vi "DM get burst by index.vi"(8 "error in (no error)":errorcluster, 10 "Burst name":i32, 11 "group":string) -> (0 "error out":errorcluster, 3 "TX burst":refnum<class "mmWave data.lvclass">)   [LabVIEW 2019, in "DataManagment.lvlib"]
uses:
  DataManagment.lvlib
  SubVIs/mmWave data_class/mmWave data.lvclass
  DM get burst by index parameters.ctl
  <vilib>/Utility/error.llb/Error Cluster From Error Code.vi
  <vilib>/ErrorRing/Error Ring.xnode
  <vilib>/addons/_JKI.lib/Serialization/JSON/JKI JSON Serialization.lvlib
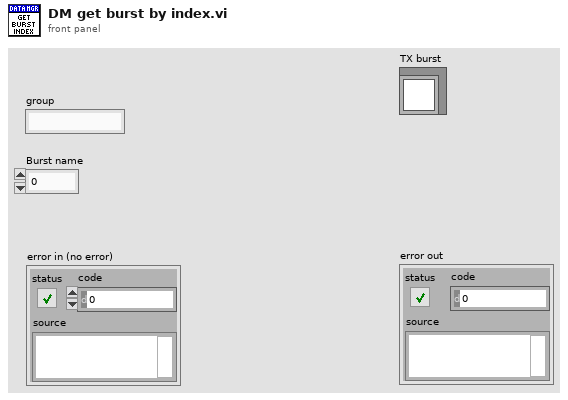
[diagram p1: front panel]
types:
  T1 = typedef "DataManagment.lvlib/DM get burst by index parameters.ctl" = cluster{"group":string, "index":i32}
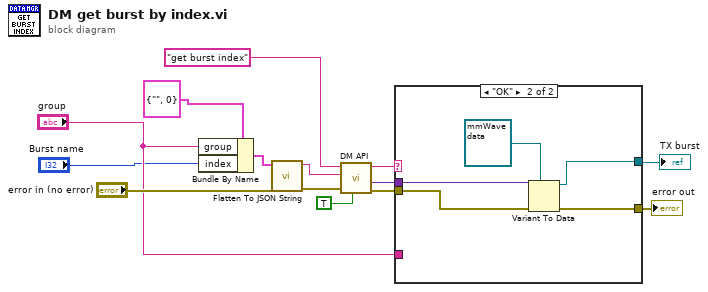
[diagram p0: block diagram]
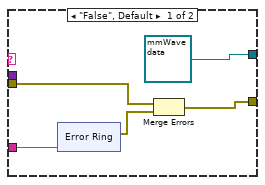
[diagram p2: hidden frame]
diagram:
  n1 = Bundle By Name(cluster=T1 {"group"="", "index"=0} ("Cluster"), "group"="group", "index"="Burst name") -> (w7:T1)
  n2 = call <vilib>:"Flatten To JSON String.vi"("error in (no error)"="error in (no error)", "Variant"=w7) -> ("error out"=w5:errorcluster, "JSON String"=w4:string)  [unwired: 8 in]
  n3 = call "DM API.vi"("response"=TRUE, "error in (no error)"=w5, "parameters"=w4, "message"="get burst index") -> ("error out"=w9:errorcluster, "data"=w11:variant, "status"=w12:string)  [unwired: 4 in, 1 out]
  n4 = case shown="\"OK\"" w12 {
    tunnel: w11 -> [_ w31]
    tunnel: [refnum<class "mmWave data.lvclass"> refnum ("mmWave data") w27] -> w10
    tunnel: [w17 w28] -> w8
    tunnel: w9 -> [w16 w29]
    tunnel: "group" -> [w15 _]
    frame "False", Default {
      n5 = xnode "Error Ring"("parameter 0"=w15) -> ("error out"=w18:errorcluster)
      n6 = Merge Errors(w16, w18) -> (w17:errorcluster)
    }
    frame "OK" {
      n7 = Variant To Data(error in=w29, type=refnum<class "mmWave data.lvclass"> refnum ("Array"), Variant=w31) -> (data=w27:refnum<class "mmWave data.lvclass">, error out=w28:errorcluster)
    }
  }
  "TX burst" <- w10
  "error out" <- w8
